vi "RT Driver VI.vi"(7 "Operation":T1, 11 "Device Reference in":T2 format="%.0x") -> (0 "Error Code":i32)   [LabVIEW 2024, in "Nominal Client Engine.lvlib"]
uses:
  Nominal Client Engine.lvlib
  <vilib>/NI VeriStand/Custom Device API/Custom Device Item Ref.ctl
  <vilib>/NI VeriStand/Custom Device API/Hardware Interface Driver VI Operation.ctl
  Shared/Compiled.Settings.ctl
  <vilib>/NI/NIVS Inline Async API/_VS Inline Async API/VS Inline Async API/VS Inline Async API.lvclass
  Streaming Specification.ctl
  Group Buffer Data.ctl
  Property Specification.ctl
  <vilib>/NI/NIVS Inline Async API/_VS Inline Async API/VS Inline Async API/VS Inline Async API.lvclass/VS Inline Async API.ctl
  <vilib>/NI/NIVS Inline Async API/_Data Access Engine/Data Access Engine/Data Access Engine.lvclass/Data Access Engine.ctl
  <vilib>/NI/NIVS Inline Async API/_Data Access Engine/Access Type Classes/Write/Write.lvclass/Write.ctl
  <vilib>/NI/NIVS Inline Async API/_Data Access Engine/Access Type Classes/ReadWrite/ReadWrite.lvclass/ReadWrite.ctl
  <vilib>/NI/NIVS Inline Async API/_Data Access Engine/Access Type Classes/Read/Read.lvclass/Read.ctl
  <vilib>/NI/NIVS Inline Async API/_Data Access Engine/Data Access Engine/Methods/Data.Engine.Read Data from HW.vi
  <vilib>/NI/NIVS Inline Async API/_VS Inline Async API/Error Handling Process/SubVIs/Error.GetError.vi
  <vilib>/NI/NIVS Inline Async API/_Data Access Engine/Data Access Engine/Methods/Data.Engine.Write Data to HW.vi
  <vilib>/NI/NIVS Inline Async API/_Data Access Engine/Access Type Classes/ReadWrite/ReadWrite.EngineData.vi
  <vilib>/NI/NIVS Inline Async API/_Data Access Engine/Access Type Classes/Write/Write.EngineData.vi
  <vilib>/NI/NIVS Inline Async API/_Data Access Engine/Access Type Classes/Read/Read.EngineData.vi
  <vilib>/NI VeriStand/Custom Device API/NI VeriStand - Get Channel Value by Data Reference.vi
  <vilib>/NI VeriStand/Custom Device API/NI VeriStand - Set Channel Value by Data Reference.vi
  <vilib>/NI VeriStand/Custom Device API/NI VeriStand - Set Channel Values by Block Data Reference.vi
  <vilib>/NI VeriStand/Custom Device API/NI VeriStand - Get Channel Values by Block Data Reference.vi
  Nominal Client.Async.vi
  Shared/Constants.vi
  <vilib>/NI VeriStand/Custom Device API/Get Item Property (Variant).vi
  <vilib>/NI VeriStand/Custom Device API/Global Data Refs.vi
  <vilib>/NI VeriStand/Custom Device API/Custom Device API.lvlib
  Shared/Nominal Client Shared.lvlib
  <vilib>/NI VeriStand/Custom Device Tools/Custom Device Utility Library/Custom Device Utility Library.lvlib
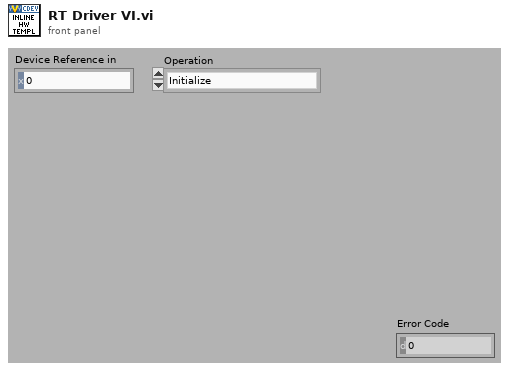
[diagram p1: front panel]
types:
  T1 = typedef "Custom Device API.lvlib/Hardware Interface Driver VI Operation.ctl" = enum16{"Initialize", "Start", "Read Data from HW", "Write Data to HW", "Close"}
  T2 = typedef "Custom Device API.lvlib/Custom Device Item Ref.ctl" = u64
  T3 = typedef "Nominal Client Shared.lvlib/Compiled.Settings.ctl" = cluster{"Name":string, "Async Init Timeout":u16, "api key":string, "datasource connection name":string, "create new datasource":bool}
  T4 = cluster{"Compiled.Settings":T3, "Async":refnum<class "VS Inline Async API.lvclass">, "error out":errorcluster}
  T5 = typedef "Nominal Client Engine.lvlib/Streaming Specification.ctl" = cluster{"Name":string, "Channels":string[], "Description":string, "Buffer Data":T6, "Channel Properties":cluster{"Array":T7[]}[], "dt":dbl}
  T6 = typedef "Nominal Client Engine.lvlib/Group Buffer Data.ctl" = cluster{"Last":i32, "Start":i32, "Length":i32, "Channel Count":i32, "Data":dbl[][], "Last Trigger":bool}
  T7 = typedef "Nominal Client Engine.lvlib/Property Specification.ctl" = cluster{"Name":string, "Value":variant}
  T8 = cluster{"Compiled.Settings":T3, "Streaming spec":T5, "Device Reference":T2}
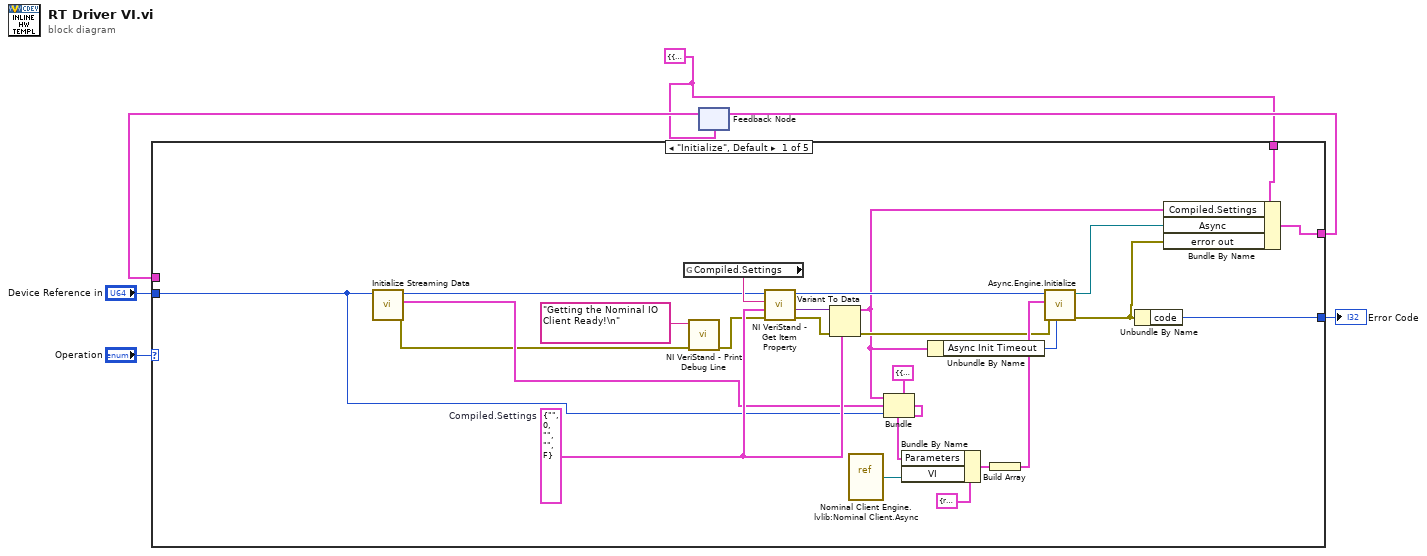
[diagram p0: block diagram]
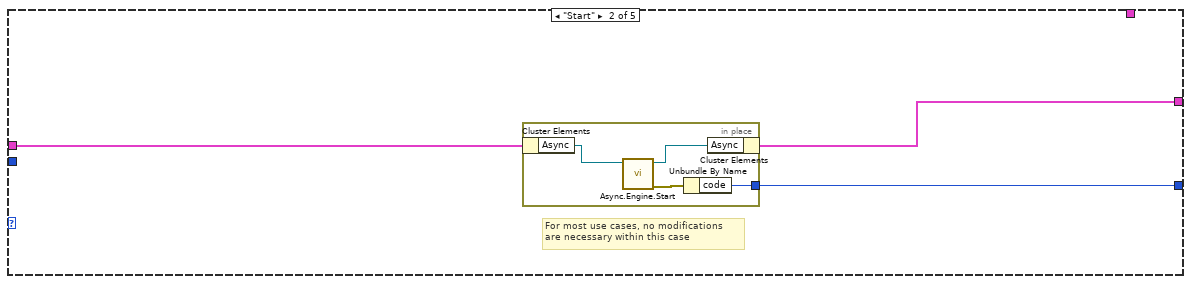
[diagram p2: hidden frame]
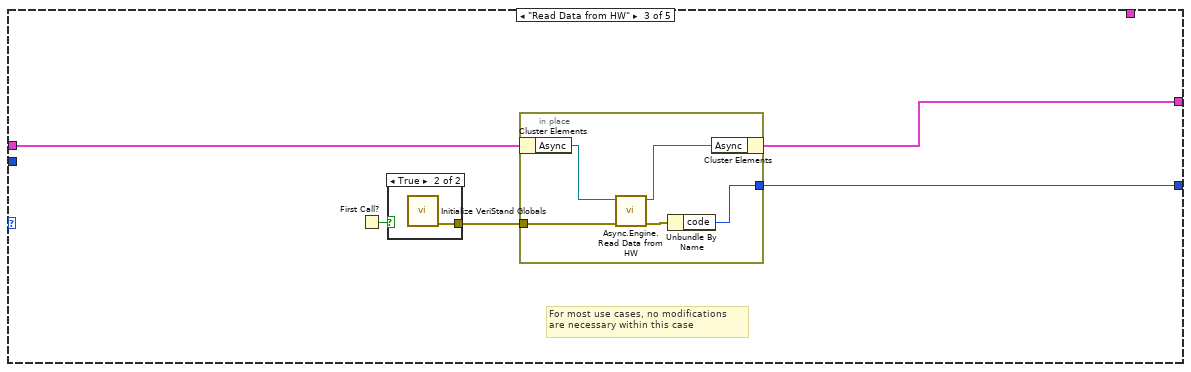
[diagram p3: hidden frame]
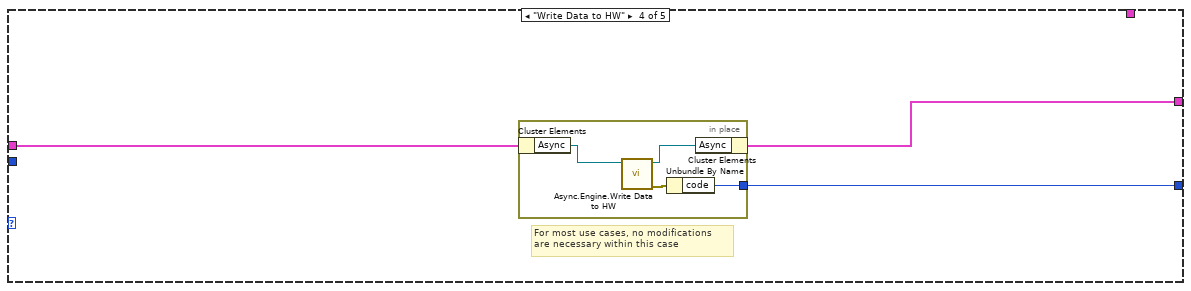
[diagram p5: hidden frame]
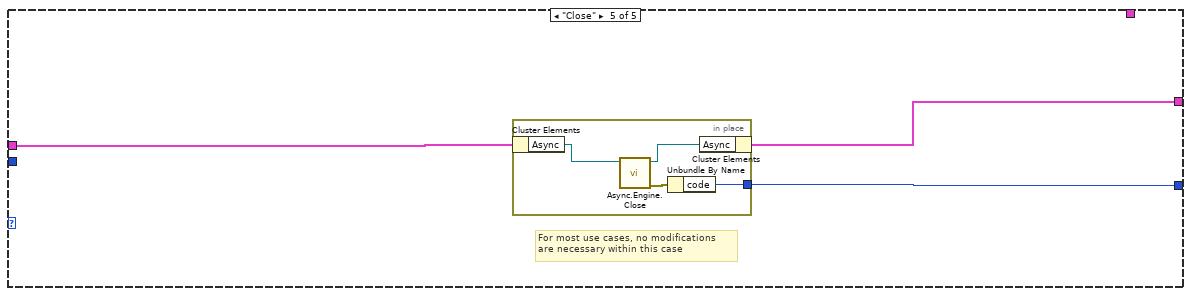
[diagram p6: hidden frame]
diagram:
  w1 = T4 {"Compiled.Settings"={"Name"="", "Async Init Timeout"=0, "api key"="", "datasource connection name"="", "create new datasource"=FALSE}, "Async"=refnum, "error out"={"status"=FALSE, "code"=0, "source"=""}} ("output cluster")
  n1 = feedback #1(w1) -> (w4:T4)
  n2 = case shown="\"Initialize\", Default" "Operation" {
    tunnel: [w30 w33 w41 w51 w59] -> w5
    tunnel: w4 -> [_ w34 w43 w50 w57]
    tunnel: "Device Reference in" -> [w7 _ _ _ _]
    tunnel: [w31 w32 w42 w52 w58] -> w2
    tunnel: w1 -> [w13 _ _ _ _]
    frame "Initialize", Default {
      w24 = T3 {"Name"="", "Async Init Timeout"=0, "api key"="", "datasource connection name"="", "create new datasource"=FALSE}  # Compiled.Settings
      n3 = call "Initialize Streaming Data.vi"("Device Ref in"=w7) -> ("error out"=w9:errorcluster, "Streaming spec"=w10:T5, "Device Ref out"=w8:T2)  [unwired: 5 in, 3 out]
      n4 = global read "Constants.vi" "Compiled.Settings"() -> (w25:string)
      n5 = call <vilib>:"NI VeriStand - Print Debug Line.vi"("error in (no error)"=w9, "Message"="Getting the Nominal IO Client Ready!\n") -> ("error out"=w17:errorcluster)  [unwired: 9 in]
      n6 = call-poly <vilib>:"NI VeriStand - Get Item Property.vi"("error in (no error)"=w17, "Default Value"=w24, "Property Name"=w25, "Item Ref in"=w8) -> ("error out"=w27:errorcluster, "Value"=w26:variant, "Item Ref out"=w21:T2)  [unwired: 4 in, 1 out]
      n7 = Variant To Data(error in=w27, type=w24, Variant=w26) -> (data=w12:T3, error out=w22:errorcluster)
      n8 = vi-ref "Nominal Client Engine.lvlib:Nominal Client.Async.vi"() -> (w20:refnum<vi>)
      n9 = Bundle(cluster=T8 {"Compiled.Settings"={"Name"="", "Async Init Timeout"=0, "api key"="", "datasource connection name"="", "create new datasource"=FALSE}, "Streaming spec"={"Name"="", "Channels"=[], "Description"="", "Buffer Data"={"Last"=0, "Start"=0, "Length"=0, "Channel Count"=0, "Data"=[], "Last Trigger"=FALSE}, "Channel Properties"=[], "dt"=0.0}, "Device Reference"=0}, "Compiled.Settings"=w12, "Streaming spec"=w10, "Device Reference"=w7) -> (w16:T8)
      n10 = Bundle By Name(cluster=cluster{"VI":refnum<vi>, "Parameters":variant} {"VI"=refnum, "Parameters"=variant} ("Process"), "Parameters"=w16, "VI"=w20) -> (w28:cluster{"VI":refnum<vi>, "Parameters":variant})
      n11 = Unbundle By Name(w12) -> ("Async Init Timeout"=w19:u16)
      n12 = Build Array(w28) -> (w23:cluster{"VI":refnum<vi>, "Parameters":variant}[])
      n13 = call <vilib>:"Async.Engine.Initialize.vi"("Timeout (ms) (5000)"=w19, "error in (no error)"=w22, "Processes"=w23, "Custom Device Ref"=w21) -> ("error out"=w11:errorcluster, "Async"=w14:refnum<class "VS Inline Async API.lvclass">)  [unwired: 6 in]
      n14 = Unbundle By Name(w11) -> ("code"=w31:i32)
      n15 = Bundle By Name(cluster=w13, "Compiled.Settings"=w12, "Async"=w14, "error out"=w11) -> (w30:T4)
    }
    frame "Start" {
      # "For most use cases, no modifications \nare necessary within this case"
      n16 = in-place {
        in-place-border: [w36] -> w32
        n17 = in-place-cluster #2(w34) -> ("Async"=w35:refnum<class "VS Inline Async API.lvclass">)
        n18 = call <vilib>:"Async.Engine.Start.vi"("VS Inline Async API in"=w35) -> ("error out"=w37:errorcluster, "VS Inline Async API out"=w38:refnum<class "VS Inline Async API.lvclass">)  [unwired: 9 in]
        n19 = Unbundle By Name(w37) -> ("code"=w36:i32)
        n20 = in-place-cluster #2("Async"=w38) -> (w33:T4)
      }
    }
    frame "Read Data from HW" {
      # "For most use cases, no modifications \nare necessary within this case"
      n21 = First Call?() -> (First Call?: T/F=w39:bool)
      n22 = case shown="True" w39 {
        tunnel: [_ w44] -> w40
        frame False {
        }
        frame True {
          n23 = call "Initialize VeriStand Globals.vi"() -> ("error out"=w44:errorcluster)  [unwired: 11 in]
        }
      }
      n24 = in-place {
        in-place-border: [w48] -> w42
        in-place-border: w40 -> [w46]
        n25 = in-place-cluster #3(w43) -> ("Async"=w45:refnum<class "VS Inline Async API.lvclass">)
        n26 = call <vilib>:"Async.Engine.Read Data from HW.vi"("error in"=w46, "Async in"=w45) -> ("error out"=w47:errorcluster, "Async out"=w49:refnum<class "VS Inline Async API.lvclass">)  [unwired: 8 in]
        n27 = Unbundle By Name(w47) -> ("code"=w48:i32)
        n28 = in-place-cluster #3("Async"=w49) -> (w41:T4)
      }
    }
    frame "Write Data to HW" {
      # "For most use cases, no modifications \nare necessary within this case"
      n29 = in-place {
        in-place-border: [w56] -> w52
        n30 = in-place-cluster #4(w50) -> ("Async"=w53:refnum<class "VS Inline Async API.lvclass">)
        n31 = call <vilib>:"Async.Engine.Write Data to HW.vi"("VS Inline Async API in"=w53) -> ("error out"=w55:errorcluster, "VS Inline Async API out"=w54:refnum<class "VS Inline Async API.lvclass">)  [unwired: 9 in]
        n32 = Unbundle By Name(w55) -> ("code"=w56:i32)
        n33 = in-place-cluster #4("Async"=w54) -> (w51:T4)
      }
    }
    frame "Close" {
      # "For most use cases, no modifications \nare necessary within this case"
      n34 = in-place {
        in-place-border: [w62] -> w58
        n35 = in-place-cluster #5(w57) -> ("Async"=w60:refnum<class "VS Inline Async API.lvclass">)
        n36 = call <vilib>:"Async.Engine.Close.vi"("Async in"=w60) -> ("error out"=w61:errorcluster, "Async out"=w63:refnum<class "VS Inline Async API.lvclass">)  [unwired: 9 in]
        n37 = Unbundle By Name(w61) -> ("code"=w62:i32)
        n38 = in-place-cluster #5("Async"=w63) -> (w59:T4)
      }
    }
  }
  "Error Code" <- w2
  n39 = feedback-in #1(w5) -> ()
